vi "Globals.vi"() -> ()   [LabVIEW 2020]
panel:
  out "NI9361CounterACTIVE":bool
  out "NI9361Counter":dbl[](array[numeric])
  out "NI9211ThermocoupleACTIVE":bool
  out "NI9211Thermocouple":dbl[](array[numeric])
  out "NI9252VOLTAGEACTIVE":bool
  out "NI9252Voltage":dbl[](array[numeric])
  out "NI9216RTDACTIVE":bool
  out "NI9216RTD":dbl[](array[numeric])
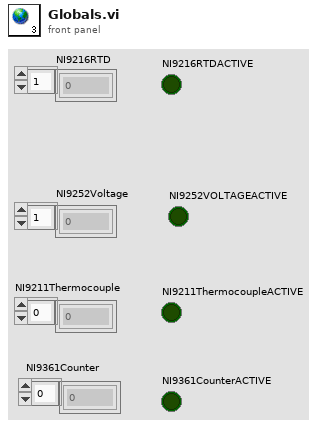
[diagram p1: front panel]
diagram:
